vi "control logic check.vi"() -> ()   [LabVIEW 2021]
panel:
  in  "stop":bool
  in  "Program Start":bool
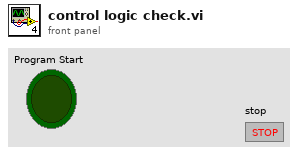
[diagram p1: front panel]
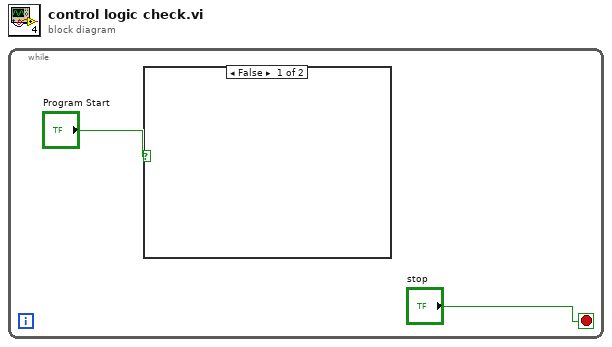
[diagram p0: block diagram]
diagram:
  n1 = while {
    stop <- "stop" stop-if-true
    n2 = case shown="False" "Program Start" {
      frame False {
      }
      frame True {
      }
    }
  }
